vi "Main.vi"(8 "error in (no error)":errorcluster, 11 "AOTFBase in":refnum<class "AOTF.lvclass">) -> (0 "error out":errorcluster, 3 "component":refnum<class "AOTF.lvclass">)   [LabVIEW 2012, in "AOTF.lvclass"]
doc: "Main VI of the component."
uses:
  AOTF.lvclass
  <vilib>/Distrio/Murmex/Murmex/command_enum.ctl
  Controls/laser line ring.ctl
  <vilib>/Distrio/Murmex/InitialiseMessage/InitialiseMessage.lvclass
  AOTF.lvclass/AOTF.ctl
  <vilib>/Distrio/Murmex/ConfigureMessage/ConfigureMessage.lvclass
  <vilib>/Distrio/Murmex/TerminateMessage/TerminateMessage.lvclass
  <vilib>/Distrio/Murmex/Murmex/update_cluster.ctl
  <vilib>/Distrio/Murmex/Murmex/Set configure at initialise.vi
  <vilib>/Distrio/Murmex/Murmex/Set VI reference.vi
  <vilib>/Distrio/Murmex/Murmex/Get ID.vi
  <vilib>/Distrio/Murmex/Murmex/Set log reference.vi
  <vilib>/Distrio/Murmex/Murmex/Set write log to disk.vi
  <vilib>/Distrio/Murmex/Murmex/Murmex.lvclass
  <vilib>/Distrio/Murmex/Message/Message.lvclass
panel:
  in  "button::configure":bool
  in  "button::quit":bool
  out "terminate?":bool=TRUE
  in  "Tab Control":enum32{"Main", "Debug"}(tab)
  in  "Power":dbl(knob) caption="Power [%]" min=0.0 max=100.0 scale=0.0..100.0
  in  "Wavelength":T1=10 items=["Blind"=10, "405nm"=0, "445nm"=5, "491nm"=1, "515nm"=2, "561nm"=3]
  out "log":string="\r\n11:11:41.970 05/12/2013: initialise from AOTF to AOTF\r\n11:11:42.586 05/12/2013: inform from AOTF to AOTF\r\n11:11:43.913 05/12/2013: update from AOTF to AOTF\r\n11:11:45.142 05/12/2013: generic (shutter_off) from AOTF to AOTF\r\n11:11:45.270 05/12/2013: generic (shutter_on) from AOTF to AOTF\r\n11:11:45.902 05/12/2013: generic (shutter_off) from AOTF to AOTF\r\n11:11:45.932 05/12/2013: inspect from AOTF to AOTF\r\n11:11:48.013 05/12/2013: configure from AOTF to AOTF\r\n11:11:52.003 05/12/2013: inform from AOTF to AOTF\r\n11:11:58.521 05/12/2013: initialise from AOTF to AOTF\r\n11:11:58.561 05/12/2013: inform from AOTF to AOTF\r\n11:11:58.695 05/12/2013: inform from AOTF to AOTF\r\n11:12:02.089 05/12/2013: update from AOTF to AOTF\r\n11:12:02.308 05/12/2013: inspect from AOTF to AOTF\r\n11:12:02.364 05/12/2013: inform from AOTF to AOTF\r\n11:12:05.062 05/12/2013: generic (shutter_on) from AOTF to AOTF\r\n11:12:06.690 05/12/2013: update from AOTF to AOTF\r\n11:12:06.909 05/12/2013: inspect from AOTF to AOTF\r\n11:12:06.964 05/12/2013: inform from AOTF to AOTF\r\n11:12:07.770 05/12/2013: update from AOTF to AOTF\r\n11:12:07.989 05/12/2013: inspect from AOTF to AOTF\r\n11:12:08.044 05/12/2013: inform from AOTF to AOTF\r\n11:12:08.627 05/12/2013: update from AOTF to AOTF\r\n11:12:08.846 05/12/2013: inspect from AOTF to AOTF\r\n11:12:08.900 05/12/2013: inform from AOTF to AOTF\r\n11:12:09.290 05/12/2013: update from AOTF to AOTF\r\n11:12:09.508 05/12/2013: inspect from AOTF to AOTF\r\n11:12:09.563 05/12/2013: inform from AOTF to AOTF\r\n11:12:10.154 05/12/2013: update from AOTF to AOTF\r\n11:12:10.373 05/12/2013: inspect from AOTF to AOTF\r\n11:12:10.430 05/12/2013: inform from AOTF to AOTF\r\n11:12:20.953 05/12/2013: update from AOTF to AOTF\r\n11:12:21.172 05/12/2013: inspect from AOTF to AOTF\r\n11:12:21.227 05/12/2013: inform from AOTF to AOTF\r\n11:12:22.057 05/12/2013: update from AOTF to AOTF\r\n11:12:22.276 05/12/2013: inspect from AOTF to AOTF\r\n11:12:22.330 05/12/2013: inform from AOTF to AOTF\r\n11:12:22.841 05/12/2013: update from AOTF to AOTF\r\n11:12:23.060 05/12/2013: inspect from AOTF to AOTF\r\n11:12:23.114 05/12/2013: inform from AOTF to AOTF\r\n11:12:23.449 05/12/2013: update from AOTF to AOTF\r\n11:12:23.668 05/12/2013: inspect from AOTF to AOTF\r\n11:12:23.724 05/12/2013: inform from AOTF to AOTF\r\n11:12:24.514 05/12/2013: update from AOTF to AOTF\r\n11:12:24.733 05/12/2013: inspect from AOTF to AOTF\r\n11:12:24.789 05/12/2013: inform from AOTF to AOTF\r\n11:12:25.098 05/12/2013: update from AOTF to AOTF\r\n11:12:25.317 05/12/2013: inspect from AOTF to AOTF\r\n11:12:25.371 05/12/2013: inform from AOTF to AOTF\r\n11:12:26.482 05/12/2013: update from AOTF to AOTF\r\n11:12:26.701 05/12/2013: inspect from AOTF to AOTF\r\n11:12:26.755 05/12/2013: inform from AOTF to AOTF\r\n11:12:27.154 05/12/2013: update from AOTF to AOTF\r\n11:12:27.373 05/12/2013: inspect from AOTF to AOTF\r\n11:12:27.428 05/12/2013: inform from AOTF to AOTF\r\n11:12:27.666 05/12/2013: update from AOTF to AOTF\r\n11:12:27.885 05/12/2013: inspect from AOTF to AOTF\r\n11:12:27.944 05/12/2013: inform from AOTF to AOTF\r\n11:12:33.380 05/12/2013: update from AOTF to AOTF\r\n11:12:33.484 05/12/2013: update from AOTF to AOTF\r\n11:12:33.603 05/12/2013: inspect from AOTF to AOTF\r\n11:12:33.611 05/12/2013: update from AOTF to AOTF\r\n11:12:33.684 05/12/2013: update from AOTF to AOTF\r\n11:12:33.740 05/12/2013: update from AOTF to AOTF\r\n11:12:33.827 05/12/2013: inspect from AOTF to AOTF\r\n11:12:33.835 05/12/2013: update from AOTF to AOTF\r\n11:12:33.897 05/12/2013: inform from AOTF to AOTF\r\n11:12:33.903 05/12/2013: update from AOTF to AOTF\r\n11:12:33.940 05/12/2013: update from AOTF to AOTF\r\n11:12:34.085 05/12/2013: update from AOTF to AOTF\r\n11:12:34.119 05/12/2013: inspect from AOTF to AOTF\r\n11:12:34.292 05/12/2013: update from AOTF to AOTF\r\n11:12:34.336 05/12/2013: inspect from AOTF to AOTF\r\n11:12:34.553 05/12/2013: inspect from AOTF to AOTF\r\n11:12:34.608 05/12/2013: inform from AOTF to AOTF\r\n11:12:34.739 05/12/2013: update from AOTF to AOTF\r\n11:12:34.771 05/12/2013: update from AOTF to AOTF\r\n11:12:34.826 05/12/2013: inspect from AOTF to AOTF\r\n11:12:34.834 05/12/2013: update from AOTF to AOTF\r\n11:12:34.867 05/12/2013: update from AOTF to AOTF\r\n11:12:34.931 05/12/2013: update from AOTF to AOTF\r\n11:12:34.979 05/12/2013: update from AOTF to AOTF\r\n11:12:35.003 05/12/2013: update from AOTF to AOTF\r\n11:12:35.027 05/12/2013: update from AOTF to AOTF\r\n11:12:35.041 05/12/2013: update from AOTF to AOTF\r\n11:12:35.051 05/12/2013: inspect from AOTF to AOTF\r\n11:12:35.066 05/12/2013: update from AOTF to AOTF\r\n11:12:35.116 05/12/2013: update from AOTF to AOTF\r\n11:12:35.171 05/12/2013: update from AOTF to AOTF\r\n11:12:35.211 05/12/2013: update from AOTF to AOTF\r\n11:12:35.273 05/12/2013: inspect from AOTF to AOTF\r\n11:12:35.287 05/12/2013: update from AOTF to AOTF\r\n11:12:35.475 05/12/2013: update from AOTF to AOTF\r\n11:12:35.495 05/12/2013: inspect from AOTF to AOTF\r\n11:12:35.549 05/12/2013: inform from AOTF to AOTF\r\n11:12:35.764 05/12/2013: inspect from AOTF to AOTF\r\n11:12:35.819 05/12/2013: inform from AOTF to AOTF\r\n11:12:35.861 05/12/2013: update from AOTF to AOTF\r\n11:12:35.877 05/12/2013: inform from AOTF to AOTF\r\n11:12:35.947 05/12/2013: update from AOTF to AOTF\r\n11:12:36.067 05/12/2013: update from AOTF to AOTF\r\n11:12:36.100 05/12/2013: inspect from AOTF to AOTF\r\n11:12:36.235 05/12/2013: update from AOTF to AOTF\r\n11:12:36.317 05/12/2013: inspect from AOTF to AOTF\r\n11:12:36.371 05/12/2013: inform from AOTF to AOTF\r\n11:12:36.587 05/12/2013: inspect from AOTF to AOTF\r\n11:12:36.771 05/12/2013: update from AOTF to AOTF\r\n11:12:36.804 05/12/2013: inspect from AOTF to AOTF\r\n11:12:37.020 05/12/2013: inspect from AOTF to AOTF\r\n11:12:37.238 05/12/2013: inspect from AOTF to AOTF\r\n11:12:37.456 05/12/2013: inspect from AOTF to AOTF\r\n11:12:37.673 05/12/2013: inspect from AOTF to AOTF\r\n11:12:37.891 05/12/2013: inspect from AOTF to AOTF\r\n11:12:37.946 05/12/2013: inform from AOTF to AOTF\r\n11:12:38.161 05/12/2013: inspect from AOTF to AOTF\r\n11:12:38.379 05/12/2013: inspect from AOTF to AOTF\r\n11:12:38.597 05/12/2013: inspect from AOTF to AOTF\r\n11:12:38.815 05/12/2013: inspect from AOTF to AOTF\r\n11:12:38.871 05/12/2013: inform from AOTF to AOTF\r\n11:12:39.086 05/12/2013: inspect from AOTF to AOTF\r\n11:12:39.303 05/12/2013: inspect from AOTF to AOTF\r\n11:12:39.363 05/12/2013: inform from AOTF to AOTF\r\n11:12:39.417 05/12/2013: inform from AOTF to AOTF\r\n11:12:39.633 05/12/2013: inspect from AOTF to AOTF\r\n11:12:39.852 05/12/2013: inspect from AOTF to AOTF\r\n11:12:40.069 05/12/2013: inspect from AOTF to AOTF\r\n11:12:40.124 05/12/2013: inform from AOTF to AOTF\r\n11:12:40.339 05/12/2013: inspect from AOTF to AOTF\r\n11:12:40.395 05/12/2013: inform from AOTF to AOTF\r\n11:12:40.448 05/12/2013: inform from AOTF to AOTF\r\n11:12:40.663 05/12/2013: inspect from AOTF to AOTF\r\n11:12:40.718 05/12/2013: inform from AOTF to AOTF\r\n11:12:40.770 05/12/2013: inform from AOTF to AOTF\r\n11:12:40.824 05/12/2013: inform from AOTF to AOTF\r\n11:12:40.877 05/12/2013: inform from AOTF to AOTF\r\n11:12:40.930 05/12/2013: inform from AOTF to AOTF\r\n11:12:40.982 05/12/2013: inform from AOTF to AOTF\r\n11:12:41.034 05/12/2013: inform from AOTF to AOTF\r\n11:12:41.092 05/12/2013: inform from AOTF to AOTF\r\n11:12:41.144 05/12/2013: inform from AOTF to AOTF\r\n11:12:41.196 05/12/2013: inform from AOTF to AOTF\r\n11:12:41.249 05/12/2013: inform from AOTF to AOTF\r\n11:12:41.307 05/12/2013: inform from AOTF to AOTF\r\n11:12:41.366 05/12/2013: inform from AOTF to AOTF\r\n11:12:41.424 05/12/2013: inform from AOTF to AOTF\r\n11:12:41.478 05/12/2013: inform from AOTF to AOTF\r\n11:12:41.533 05/12/2013: inform from AOTF to AOTF\r\n11:12:41.589 05/12/2013: inform from AOTF to AOTF\r\n11:12:42.246 05/12/2013: terminate from AOTF to AOTF"
  in  "component ID":string="AOTF"
  in  "button::send":bool
  in  "command":T2
  in  "Generic command":string
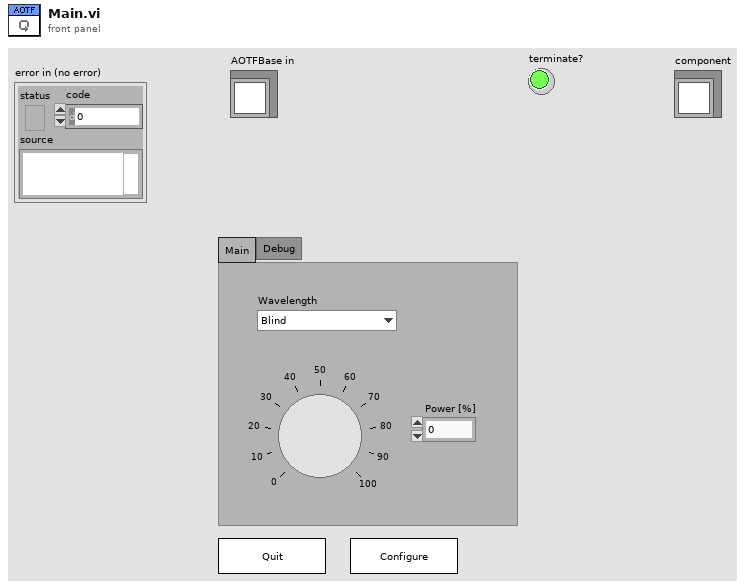
[diagram p1: front panel]
types:
  T1 = typedef "AOTF.lvclass/laser line ring.ctl" = u8
  T2 = typedef "Murmex.lvlib/Murmex.lvclass/command_enum.ctl" = enum16{"null", "initialise", "reset", "terminate", "acknowledge", "update", "inspect", "inform", "proceed", "start", "stop", "fetch", "configure", "generic"}
  T3 = enum8{"Enabled", "Disabled", "Disabled and Grayed Out"}
  T4 = typedef "Murmex.lvlib/Murmex.lvclass/update_cluster.ctl" = cluster{"target ID":string, "key chains":string[], "values":variant[]}
  T5 = typedef "Murmex.lvclass/command_enum.ctl" = enum16{"null", "initialise", "reset", "terminate", "acknowledge", "update", "inspect", "inform", "proceed", "start", "stop", "fetch", "configure", "generic"}
  T6 = typedef "Murmex.lvclass/Event type enumerations.ctl" = enum16{"before", "after"}
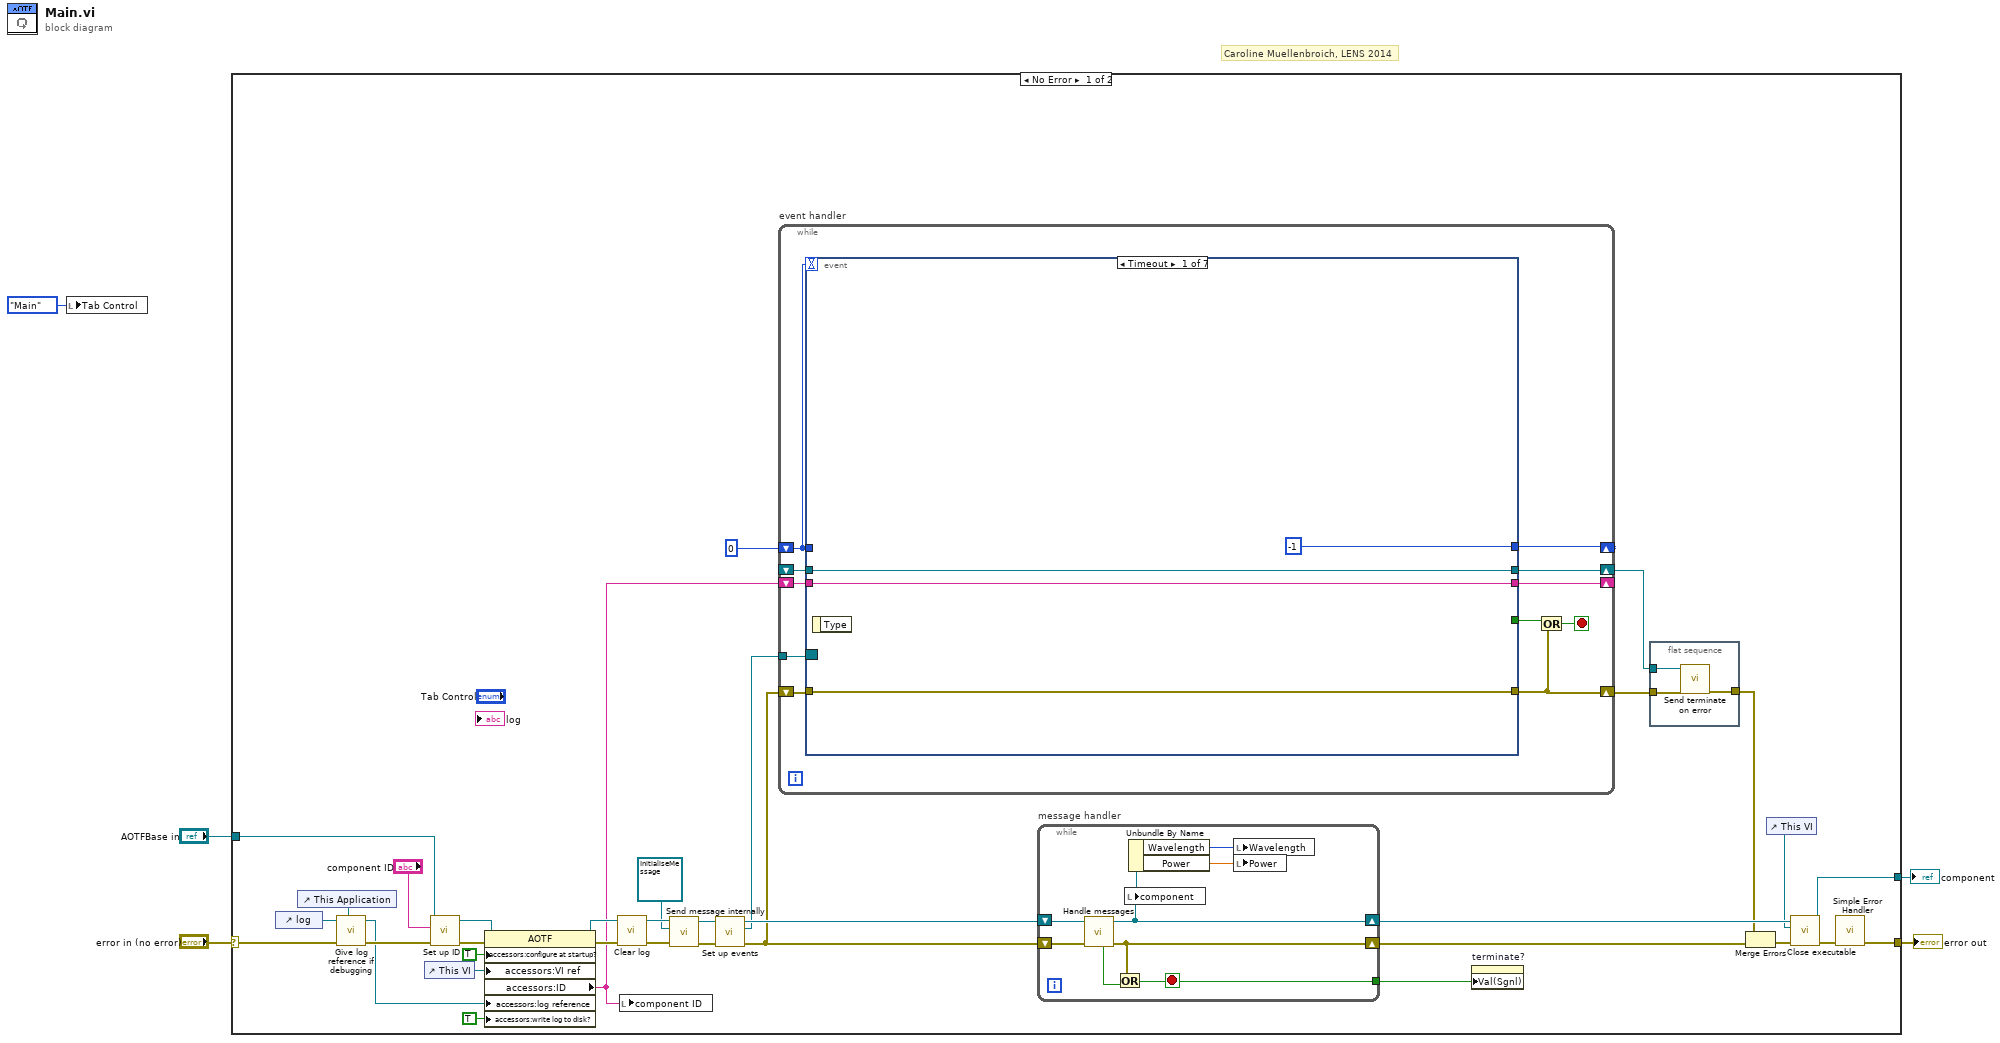
[diagram p0: block diagram]
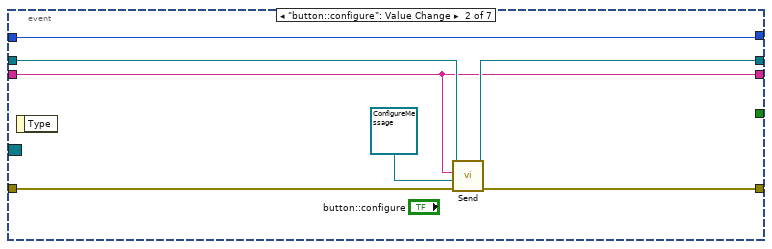
[diagram p2: hidden frame]
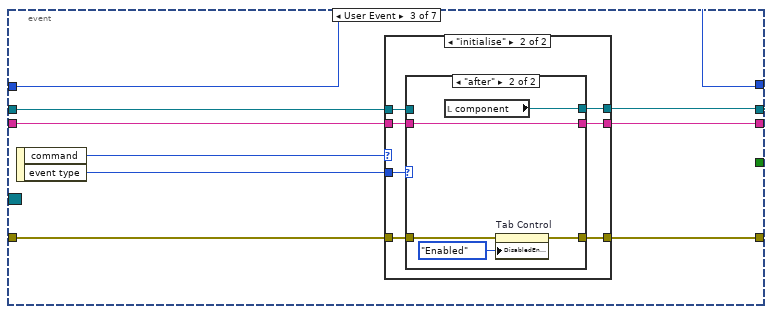
[diagram p3: hidden frame]
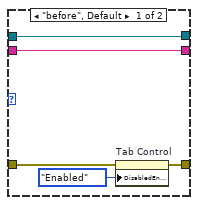
[diagram p5: hidden frame]
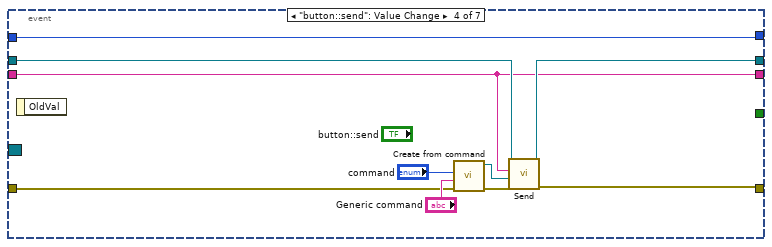
[diagram p6: hidden frame]
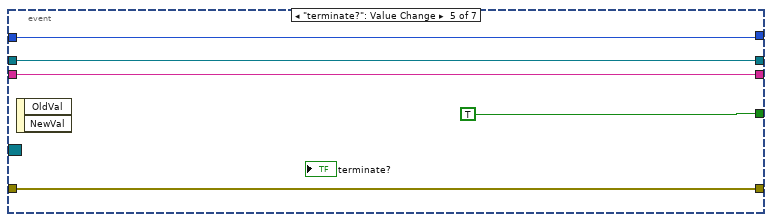
[diagram p7: hidden frame]
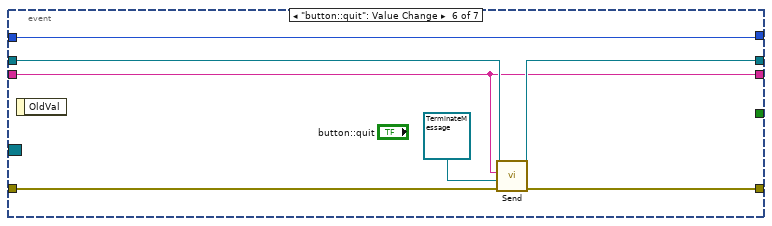
[diagram p8: hidden frame]
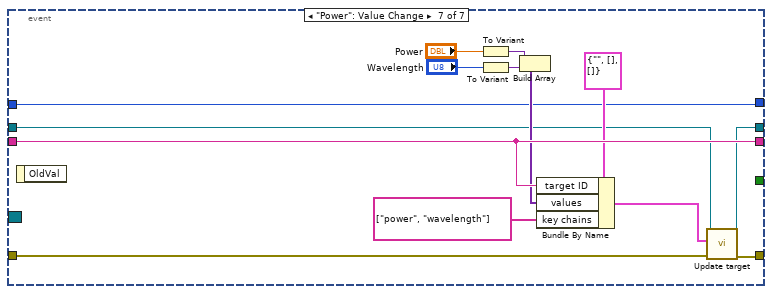
[diagram p9: hidden frame]
diagram:
  # "Caroline Muellenbroich, LENS 2014"
  n1 = local write "Tab Control"(enum32{"Main", "Debug"}."Main" ("Tab Control")) -> ()
  n2 = case shown="No Error" "error in (no error)" {
    selector: "error in (no error)" -> [w10 w140]
    tunnel: "AOTFBase in" -> [w40 w139]
    tunnel: [w25 w139] -> w5
    tunnel: [w21 w140] -> w4
    frame No Error {
      n3 = control-ref of="log"() -> (w11:refnum<vi>)
      n4 = control-ref of="This Application"() -> (w12:refnum<vi>)
      n5 = call "Give log reference if debugging.vi"("application ref"=w12, "error in (no error)"=w10, "log reference in"=w11) -> ("error out"=w9:errorcluster, "log reference out"=w8:refnum<vi>)  [unwired: 6 in, 1 out]
      n6 = control-ref of="This VI"() -> (w36:refnum<vi>)
      n7 = call <vilib>:"Set up ID.vi"("error in (no error)"=w9, "component ID"="component ID", "MurmexBase in"=w40) -> ("error out"=w39:errorcluster, "MurmexBase out"=w38:refnum<class "AOTF.lvclass">)  [unwired: 6 in, 1 out]
      n8 = property class="AOTF"(reference=w38, error in=w39, "accessors:configure at startup?"=TRUE ("configure at startup?"), "accessors:VI ref"=w36, "accessors:log reference"=w8, "accessors:write log to disk?"=TRUE ("write log to disk?")) -> (reference out=w33:refnum<class "AOTF.lvclass">, error out=w35:errorcluster, "accessors:ID"=w15:string)
      n9 = call <vilib>:"Clear log.vi"("error in (no error)"=w35, "MurmexBase in"=w33) -> ("error out"=w34:errorcluster, "MurmexBase out"=w32:refnum<class "AOTF.lvclass">)  [unwired: 8 in]
      n10 = local write "component ID"(w15) -> ()
      n11 = call <vilib>:"Send message internally.vi"("error in (no error)"=w34, "Message"=refnum<class "InitialiseMessage.lvclass"> refnum ("Murmex.lvlib:InitialiseMessage"), "Murmex in"=w32) -> ("error out"=w31:errorcluster, "Murmex out"=w7:refnum<class "AOTF.lvclass">)  [unwired: 7 in]
      n12 = call <vilib>:"Set up events.vi"("error in (no error)"=w31, "MurmexBase in"=w7) -> ("error out"=w24:errorcluster, "Event Registration Refnum"=w23:refnum<event-registration>, "MurmexBase out"=w30:refnum<class "AOTF.lvclass">)  [unwired: 7 in]
      n13 = while "event handler" {
        tunnel: w23 -> [w54]
        shift-right: [w47] -> w19
        shift-left: w24 -> [w53]
        shift-right: [w49] -> _
        shift-left: w15 -> [w52]
        shift-right: [w51] -> w17
        shift-left: _ -> [w50]
        shift-right: [w45] -> _
        shift-left: 0 -> [w44]
        stop <- w48 stop-if-true
        n14 = event shown="[0] Timeout" {
          selector: w54 -> [_ _ _ _ _ _ _]
          dyn-events: _ -> [_ _ _ _ _ _ _]
          timeout: w44 -> [_ _ _ _ _ _ _]
          tunnel: w53 -> [w56 w65 w72 w101 w109 w116 w129]
          tunnel: [w56 w64 w71 w100 w109 w115 w130] -> w47
          tunnel: w52 -> [w58 w60 w70 w96 w107 w111 w128]
          tunnel: [w57 w62 w69 w98 w106 w113 w123] -> w51
          tunnel: w50 -> [w57 w63 w68 w99 w106 w114 w119]
          tunnel: [w58 w60 w67 w96 w107 w111 w128] -> w49
          tunnel: [_ _ _ _ TRUE _ _] -> w46
          tunnel: w44 -> [_ w61 w66 w97 w105 w112 w120]
          tunnel: [-1 w61 w66 w97 w105 w112 w120] -> w45
          event Timeout {
            n15 = event-data() -> ()  [unwired: 1 in, 1 out]
          }
          event "button::configure": Value Change {
            n16 = event-data() -> ()  [unwired: 1 in, 1 out]
            n17 = call <vilib>:"Send.vi"("error in (no error)"=w65, "Message"=refnum<class "ConfigureMessage.lvclass"> refnum ("Murmex.lvlib:ConfigureMessage"), "recipient"=w60, "Murmex in"=w63) -> ("error out"=w64:errorcluster, "Murmex out"=w62:refnum<class "AOTF.lvclass">)  [unwired: 6 in]
          }
          event User Event {
            n18 = event-data() -> ("command"=w74:T5, "event type"=w73:T6)  [unwired: 1 in]
            n19 = case shown="\"initialise\"" w74 {
              tunnel: w73 -> [_ w84]
              tunnel: w72 -> [w75 w83]
              tunnel: [w75 w82] -> w71
              tunnel: w70 -> [w77 w81]
              tunnel: [w76 w80] -> w69
              tunnel: w68 -> [w76 w79]
              tunnel: [w77 w78] -> w67
              frame "null", Default {
              }
              frame "initialise" {
                n20 = case shown="\"after\"" w84 {
                  tunnel: [w88 w93] -> w82
                  tunnel: w83 -> [w89 w94]
                  tunnel: w81 -> [w86 w91]
                  tunnel: [w85 w90] -> w80
                  tunnel: w79 -> [w85 _]
                  tunnel: [w86 w91] -> w78
                  frame "before", Default {
                    n21 = property on="Tab Control" class="TabCtl (strict)"(error in=w89, "DisabledEnum"=T3."Enabled" ("Disabled")) -> (error out=w88:errorcluster)  [unwired: 1 in, 1 out]
                  }
                  frame "after" {
                    n22 = local read "component"() -> (w90:refnum<class "AOTF.lvclass">)
                    n23 = property on="Tab Control" class="TabCtl (strict)"(error in=w94, "DisabledEnum"=T3."Enabled" ("Disabled")) -> (error out=w93:errorcluster)  [unwired: 1 in, 1 out]
                  }
                }
              }
            }
          }
          event "button::send": Value Change {
            n24 = event-data() -> ()  [unwired: 1 in, 1 out]
            n25 = call <vilib>:"Create from command.vi"("error in (no error)"=w101, "generic command"="Generic command", "command"="command") -> ("error out"=w103:errorcluster, "Message out"=w102:refnum<class "Message.lvclass">)  [unwired: 7 in]
            n26 = call <vilib>:"Send.vi"("error in (no error)"=w103, "Message"=w102, "recipient"=w96, "Murmex in"=w99) -> ("error out"=w100:errorcluster, "Murmex out"=w98:refnum<class "AOTF.lvclass">)  [unwired: 6 in]
          }
          event "terminate?": Value Change {
            n27 = event-data() -> ()  [unwired: 1 in, 2 out]
          }
          event "button::quit": Value Change {
            n28 = event-data() -> ()  [unwired: 1 in, 1 out]
            n29 = call <vilib>:"Send.vi"("error in (no error)"=w116, "Message"=refnum<class "TerminateMessage.lvclass"> refnum ("Murmex.lvlib:TerminateMessage"), "recipient"=w111, "Murmex in"=w114) -> ("error out"=w115:errorcluster, "Murmex out"=w113:refnum<class "AOTF.lvclass">)  [unwired: 6 in]
          }
          event "Power": Value Change {
            n30 = event-data() -> ()  [unwired: 1 in, 1 out]
            n31 = To Variant(anything="Power") -> (Variant=w122:variant)
            n32 = To Variant(anything="Wavelength") -> (Variant=w121:variant)
            n33 = Build Array(w122, w121) -> (w124:variant[])
            n34 = Bundle By Name(cluster=T4 {"target ID"="", "key chains"=[], "values"=[]} ("update cluster"), "target ID"=w128, "values"=w124, "key chains"=string[] ["power", "wavelength"]) -> (w127:T4)
            n35 = call <vilib>:"Update target.vi"("error in (no error)"=w129, "update cluster"=w127, "MurmexBase in"=w119) -> ("error out"=w130:errorcluster, "MurmexBase out"=w123:refnum<class "AOTF.lvclass">)  [unwired: 7 in]
          }
        }
        n36 = Or(x=w46, y=w47) -> (x .or. y?=w48:bool)
      }
      n37 = while "message handler" {
        shift-right: [w133] -> w26
        shift-left: w30 -> [w137]
        shift-right: [w136] -> w27
        shift-left: w24 -> [w138]
        tunnel: [w134] -> w22
        stop <- w134 stop-if-true
        n38 = call <vilib>:"Handle messages.vi"("error in (no error)"=w138, "Murmex in"=w137) -> ("error out"=w136:errorcluster, "Murmex out"=w133:refnum<class "AOTF.lvclass">, "terminated?"=w135:bool)  [unwired: 7 in]
        n39 = Or(x=w136, y=w135) -> (x .or. y?=w134:bool)
        n40 = local write "component"(w133) -> ()
        n41 = Unbundle By Name(w133) -> ("Wavelength"=w131:T1, "Power"=w132:dbl)
        n42 = local write "Wavelength"(w131) -> ()
        n43 = local write "Power"(w132) -> ()
      }
      n44 = property on="terminate?" class="Bool (strict)"("Val(Sgnl)"=w22) -> ()  [unwired: 2 in, 2 out]
      n45 = flat-sequence {
        tunnel: w19 -> [w42]
        tunnel: [w43] -> w18
        tunnel: w17 -> [w41]
        frame #0 {
          n46 = call <vilib>:"Send terminate on error.vi"("error in (no error)"=w42, "Murmex in"=w41) -> ("error out"=w43:errorcluster)  [unwired: 8 in, 1 out]
        }
      }
      n47 = Merge Errors(w18, w27) -> (w28:errorcluster)
      n48 = control-ref of="This VI"() -> (w16:refnum<vi>)
      n49 = call <vilib>:"Close executable.vi"("error in (no error)"=w28, "main VI ref (optional)"=w16, "MurmexBase in"=w26) -> ("error out"=w29:errorcluster, "MurmexBase out"=w25:refnum<class "AOTF.lvclass">)  [unwired: 7 in]
      n50 = call <vilib>:"Simple Error Handler.vi"("error in (no error)"=w29) -> ("error out"=w21:errorcluster)  [unwired: 4 in, 4 out]
    }
    frame Error {
    }
  }
  "error out" <- w4
  "component" <- w5
